vi "Spectrograph_logEvent_reportedDisperserPosition.vi"(8 "error in (no error)":errorcluster, 11 "logevent_reportedDisperserPosition_Ctl":T1) -> (0 "error out":errorcluster, 2 "function return":i32, 3 "logevent_reportedDisperserPosition_Ctl out":T1)   [LabVIEW 2016, in "SALLV_Spectrograph.lvlib"]
doc: "int Spectrograph_shm_logEvent_reportedDisperserPositionLV(Spectrograph_logevent_reportedDisperserPositionLV *logevent_reportedDisperserPosition_Ctl );"
uses:
  SALLV_Spectrograph.lvlib
  DataTypes/logevent_reportedDisperserPosition.ctl
  SALLV_Spectrograph.so
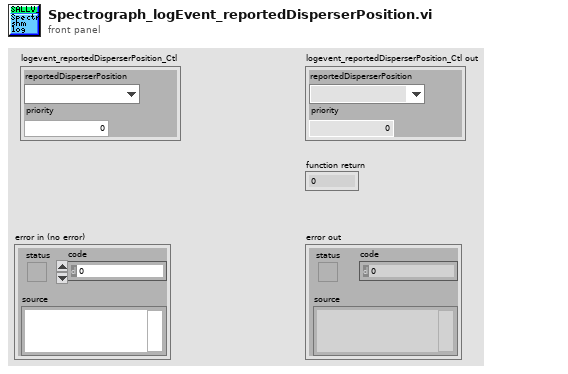
[diagram p1: front panel]
types:
  T1 = typedef "SALLV_Spectrograph.lvlib/logevent_reportedDisperserPosition.ctl" = cluster{"reportedDisperserPosition":enum32{"", "disperser0", "disperser1", "disperser2", "disperser3", "disperser4"}, "priority":i32}
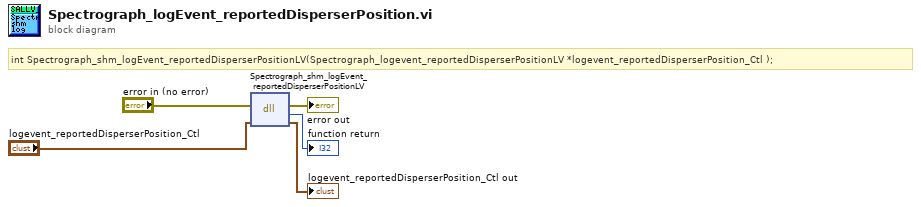
[diagram p0: block diagram]
diagram:
  # "int Spectrograph_shm_logEvent_reportedDisperserPositionLV(Spectrograph_logevent_reportedDisperserPositionLV *logevent_reportedDisperserPosition_Ctl );"
  n1 = dll-call lib="home/harini/TCS/SALLV_Spectrograph/SALLV_Spectrograph.*" fn="Spectrograph_shm_logEvent_reportedDisperserPositionLV"(error in="error in (no error)", "logevent_reportedDisperserPosition_Ctl"="logevent_reportedDisperserPosition_Ctl") -> (error out=→"error out":errorcluster, →"function return":i32, "logevent_reportedDisperserPosition_Ctl"=→"logevent_reportedDisperserPosition_Ctl out":T1)  [unwired: 2 in, 1 out]
